vi "Create VI Override.vi"(8 "error in (no error)":errorcluster, 10 "Child class":refnum<vi>, 11 "Parent Method VI":refnum<vi>) -> (0 "error out":errorcluster)   [LabVIEW 2019, in "gRPC Template Creation Utility.lvlib"]
uses:
  gRPC Template Creation Utility.lvlib
  <resource>/Framework/Providers/LVClassLibrary/NewAccessors/MemberVICreation.lvlib
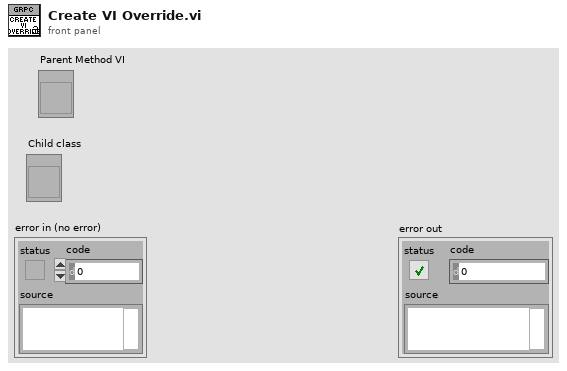
[diagram p1: front panel]
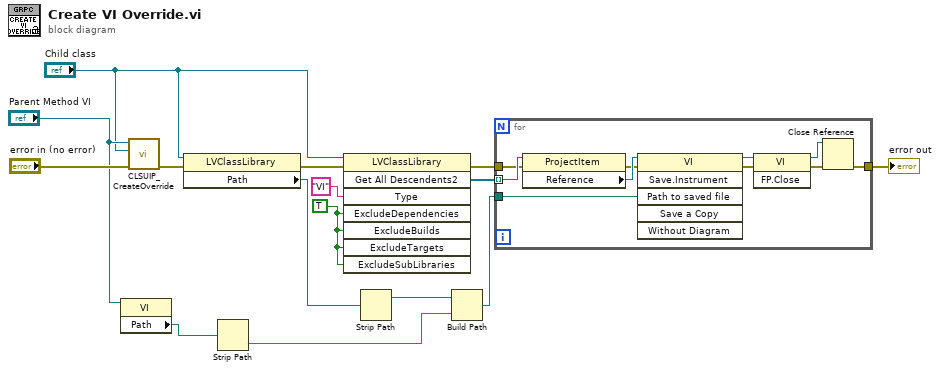
[diagram p0: block diagram]
diagram:
  w11 = TRUE ("ExcludeDependencies")
  n1 = property class="VI"(reference="Parent Method VI") -> ("Path"=w2:path)  [unwired: 1 in, 2 out]
  n2 = call <resource>:"CLSUIP_CreateOverride.vi"("error in (no error)"="error in (no error)", "Child class"="Child class", "Parent Method"="Parent Method VI") -> ("error out"=w6:errorcluster)  [unwired: 5 in, 3 out]
  n3 = property class="LVClassLibrary"(reference="Child class", error in=w6) -> (error out=w5:errorcluster, "Path"=w13:path)  [unwired: 1 out]
  n4 = Strip Path(path=w2) -> (name=w1:string)  [unwired: 1 out]
  n5 = invoke class="LVClassLibrary" method="Get All Descendents2"(reference="Child class", error in=w5, "Type"="VI", "ExcludeDependencies"=w11, "ExcludeBuilds"=w11, "ExcludeTargets"=w11, "ExcludeSubLibraries"=w11) -> (error out=w4:errorcluster, "Get All Descendents2"=w9:refnum<vi>[])  [unwired: 1 in, 6 out]
  n6 = Strip Path(path=w13) -> (stripped path=w12:path)  [unwired: 1 out]
  n7 = Build Path(base path=w12, name or relative path=w1) -> (appended path=w8:path)
  n8 = for {
    tunnel: w9 -> [w25] mode=indexing
    tunnel: w8 -> [w21]
    tunnel: w4 -> [w20]
    tunnel: [w16] -> w3
    n9 = property class="ProjectItem"(reference=w25, error in=w20) -> (error out=w19:errorcluster, "Reference"=w24:refnum<vi>)  [unwired: 1 out]
    n10 = invoke class="VI" method="Save.Instrument"(reference=w24, error in=w19, "Path to saved file"=w21) -> (reference out=w23:refnum<vi>, error out=w18:errorcluster)  [unwired: 3 in, 4 out]
    n11 = invoke class="VI" method="FP.Close"(reference=w23, error in=w18) -> (reference out=w22:refnum<vi>, error out=w17:errorcluster)  [unwired: 1 in, 1 out]
    n12 = Close Reference(reference=w22, error in (no error)=w17) -> (error out=w16:errorcluster)
  }
  "error out" <- w3
